vi "Main RT.vi"() -> ()   [LabVIEW 2025]
uses:
  <vilib>/NI_Real-Time Target Support.lvlib
  <vilib>/ptbypt/NI_PtbyPt.lvlib
panel:
  out "Signal":dbl(graph)
  in  "Frequency":dbl min=0.0
  # "Example UI Running on cRIO"
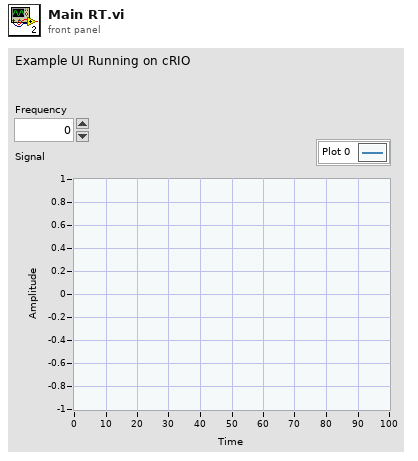
[diagram p1: front panel]
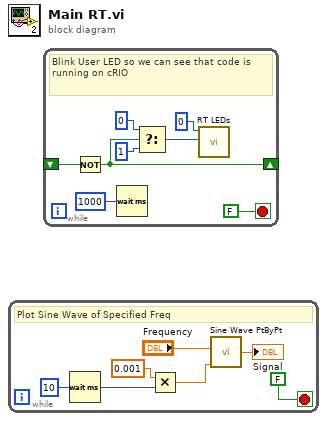
[diagram p0: block diagram]
diagram:
  n1 = while {
    stop <- FALSE ("Stop") stop-if-true
    # "Plot Sine Wave of Specified Freq"
    n2 = Wait (ms)(milliseconds to wait=u32 10) -> (millisecond timer value=w4:u32)
    n3 = Multiply(x=0.001, y=w4) -> (x*y=w2:dbl)
    n4 = call <vilib>:"Sine Wave PtByPt.vi"("time"=w2, "frequency"="Frequency") -> ("sine wave"=→"Signal":dbl)  [unwired: 2 in]
  }
  n5 = while {
    shift-right: [w10] -> _
    shift-left: _ -> [w9]
    stop <- FALSE stop-if-true
    # "Blink User LED so we can see that code is running on cRIO"
    n6 = Not(x=w9) -> (.not. x?=w10:bool)
    n7 = Wait (ms)(milliseconds to wait=u32 1000) -> ()  [unwired: 1 out]
    n8 = Select(t=0 ("State"), s=w10, f=1 ("State")) -> (s? t:f=w11:i32)
    n9 = call <vilib>:"RT LEDs.vi"("State"=w11, "LED Num"=0) -> ()  [unwired: 4 in, 2 out]
  }
